vi "Write Sweep (V_A).vi"(10 "Sweep (V/A)":string="3.3", 11 "Power Supply in":refnum<class "Power Supply.lvclass">) -> (3 "Power Supply out":refnum<class "Power Supply.lvclass">)   [LabVIEW 2020, in "Power Supply.lvclass"]
uses:
  Power Supply.lvclass
  Power Supply.lvclass/Power Supply.ctl
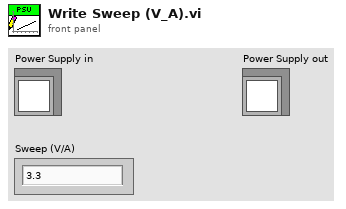
[diagram p1: front panel]
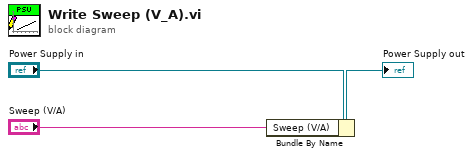
[diagram p0: block diagram]
diagram:
  n1 = Bundle By Name(cluster="Power Supply in", "Sweep (V/A)"="Sweep (V/A)") -> (→"Power Supply out":refnum<class "Power Supply.lvclass">)
